vi "Fit.vi"(8 "error in (no error)":errorcluster caption="entrée d'erreur (pas d'erreur)", 9 "y":string[][](array[string]), 10 "X":string[][](array[string]), 11 "PolynomialFeatures.lvclass":refnum<class "PolynomialFeatures.lvclass">) -> (0 "error out":errorcluster caption="sortie d'erreur", 2 "String Data":string, 3 "PolynomialFeatures.lvclass":refnum<class "PolynomialFeatures.lvclass">)   [LabVIEW 2020, in "PolynomialFeatures.lvclass"]
doc: "Compute number of output features.\n\nReturns : \n\n- String : OK"
uses:
  PolynomialFeatures.lvclass
  PolynomialFeatures.lvclass/PolynomialFeatures.ctl
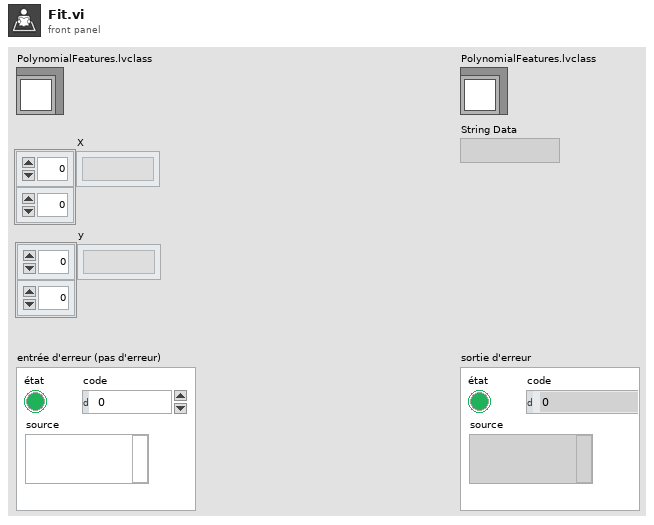
[diagram p1: front panel]
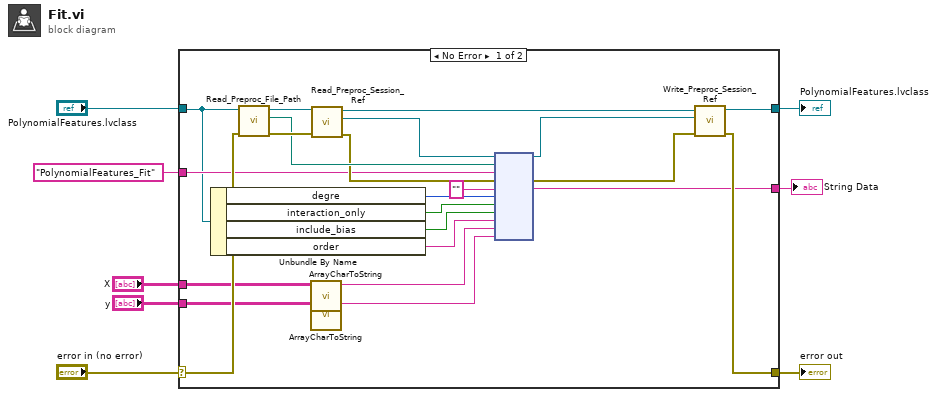
[diagram p0: block diagram]
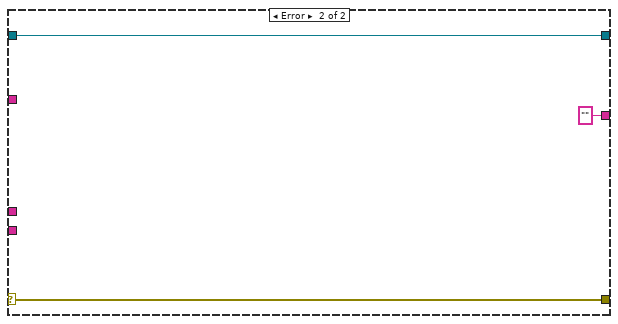
[diagram p2: hidden frame]
diagram:
  n1 = case shown="No Error" "error in (no error)" {
    selector: "error in (no error)" -> [w17 w34]
    tunnel: [w18 w34] -> w7
    tunnel: [w19 w33] -> w5
    tunnel: "PolynomialFeatures.lvclass" -> [w14 w33]
    tunnel: "PolynomialFeatures_Fit" ("Fonction") -> [w16 _]
    tunnel: [w15 ""] -> w3
    tunnel: "X" -> [w12 _]
    tunnel: "y" -> [w11 _]
    frame No Error {
      n2 = Unbundle By Name(w14) -> ("degre"=w22:i32, "interaction_only"=w21:bool, "include_bias"=w20:bool, "order"=w13:string)
      n3 = call-dynamic "Read_Preproc_File_Path.vi"("error in (no error)"=w17, "Python in"=w14) -> ("error out"=w30:errorcluster, "File_Path"=w27:path, "Python out"=w31:refnum<class "PolynomialFeatures.lvclass">)  [unwired: 7 in]
      n4 = call "ArrayCharToString.vi"("TAB"=w12) -> ("Instruction"=w10:string)  [unwired: 10 in]
      n5 = call "ArrayCharToString.vi"("TAB"=w11) -> ("Instruction"=w9:string)  [unwired: 10 in]
      n6 = call-dynamic "Read_Preproc_Session_Ref.vi"("error in (no error)"=w30, "Python in"=w31) -> ("error out"=w26:errorcluster, "Session_ref"=w28:refnum<k35>, "Python out"=w29:refnum<class "PolynomialFeatures.lvclass">)  [unwired: 7 in]
      n7 = node(w28, w27, w16, w26, "", w22, w21, w20, w13, w10, w9) -> (w24:refnum<k35>, w25:errorcluster, w15:string)  [unwired: 6 in, 2 out]
      n8 = call-dynamic "Write_Preproc_Session_Ref.vi"("error in (no error)"=w25, "Session_ref"=w24, "Python in"=w29) -> ("error out"=w18:errorcluster, "Python out"=w19:refnum<class "PolynomialFeatures.lvclass">)  [unwired: 7 in]
    }
    frame Error {
    }
  }
  "error out" <- w7
  "PolynomialFeatures.lvclass" <- w5
  "String Data" <- w3
